vi "kvCanRequestBusStatistics.vi"(2 "error in (no error)":errorcluster, 3 "Channel Handle (input only)":i32) -> (0 "error out":errorcluster, 1 "Channel Handle (output only)":i32)   [LabVIEW 2022 SP3]
doc: "The canRequestBusStatistics function requests bus staistics from the hardware. The bus statistics figures can be retrieved later by a call to the canGetBusStatistics function.\n\nNotes\nThe time between a call to canRequestBusStatistics and the point in time where the bus statistics is actually available via a call to canGetBusStatistics is not defined. Typically, you would call canRequestBusStatistics from your application periodically (for example, once per second) to request the data from the driver and then call canGetBusStatistics with the same rate to obtain the latest reported data."
uses:
  canlib32.dll
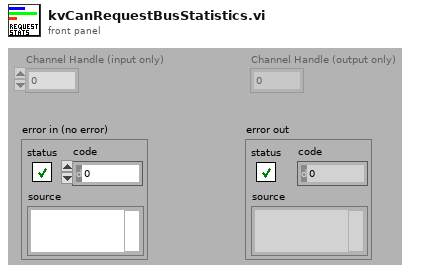
[diagram p1: front panel]
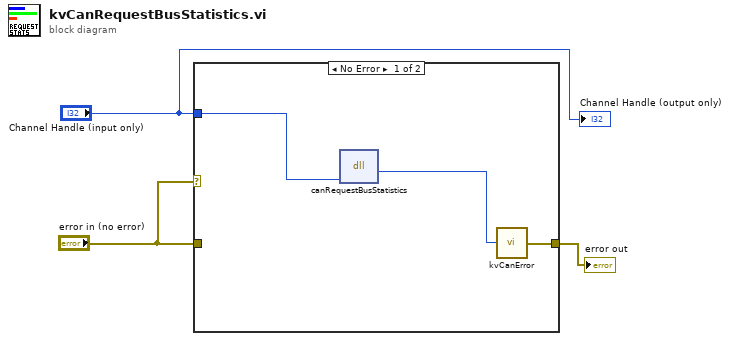
[diagram p0: block diagram]
diagram:
  n1 = case shown="No Error" "error in (no error)" {
    tunnel: "error in (no error)" -> [_ w7]
    tunnel: [w6 w7] -> w2
    tunnel: "Channel Handle (input only)" -> [w5 _]
    frame No Error {
      n2 = dll-call lib="canlib32.dll" fn="canRequestBusStatistics"("channelHandle"=w5) -> (w4:i32)  [unwired: 4 in, 2 out]
      n3 = call "kvCanError.vi"("error code"=w4) -> ("error out"=w6:errorcluster)
    }
    frame Error {
    }
  }
  "error out" <- w2
  "Channel Handle (output only)" <- "Channel Handle (input only)"
